vi "newposition.vi"(0 "x_modify":dbl, 4 "cur_y":dbl, 5 "r":dbl, 6 "cur_x":dbl, 7 "y_modify":dbl, 8 "dt":dbl=0.02, 9 "V_right":dbl, 10 "V_left":dbl, 11 "cur_angle":dbl) -> (1 "new_y":dbl, 2 "new_x":dbl, 3 "new_angle":dbl)   [LabVIEW 2015]
uses:
  Documents/LabVIEW Data/MathScriptVIs/MCStatic_35241984432_abfa35976836e38269e549687f4c5e7d.vi
  <instcachedir>/0/MCStatic_35241984432_abfa35976836e38269e549687f4c5e7d_C7C269247EEA4349BB5C711C73CDF5A1.lvgen/MCStatic_35241984432_abfa35976836e38269e549687f4c5e7d_C7C269247EEA4349BB5C711C73CDF5A1_000.vi
  <vilib>/imath/engines/lvmath2/RunTimeEngine/NodeEndStatement/NIMS_NodeEndStatement_Output.vi
  <instcachedir>/0/NIMS_NodeEndStatement_Output_53EC0D466D134D7ABD903AC30B43404B.lvgen/NIMS_NodeEndStatement_Output_53EC0D466D134D7ABD903AC30B43404B_001.vi
  <vilib>/imath/engines/lvmath2/RunTimeEngine/ErrorHandling/NIMS_Finalize Error.vi
  Documents/LabVIEW Data/Coordinates.m
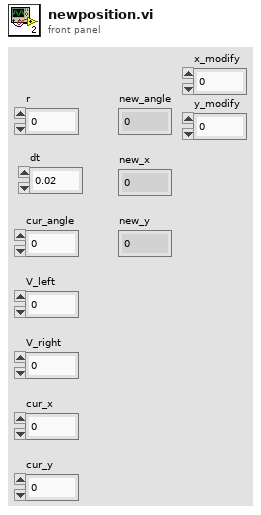
[diagram p1: front panel]
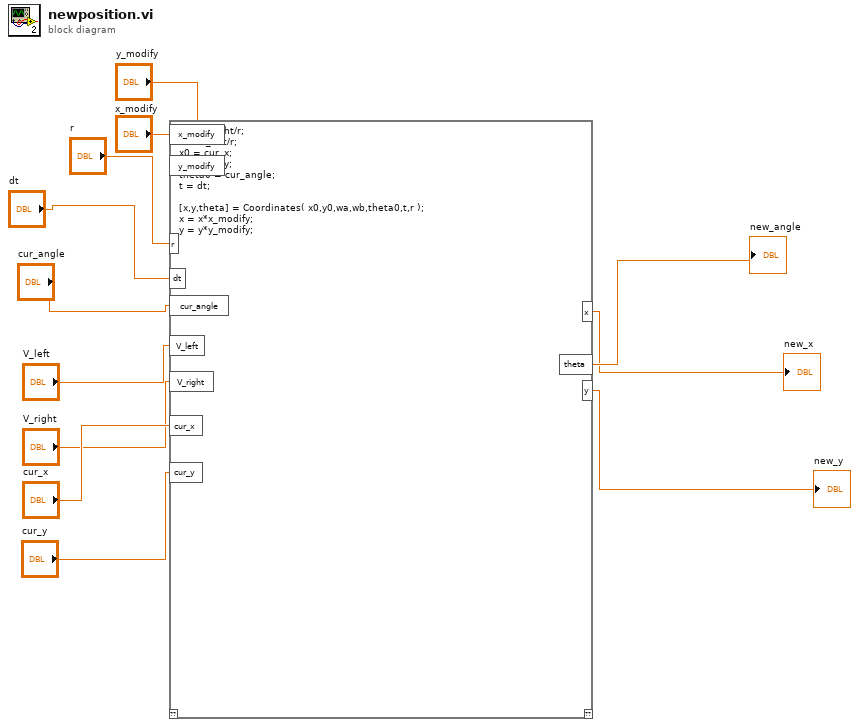
[diagram p0: block diagram]
diagram:
  n1 = mathscript code="wa=V_right/r;\nwb=V_left/r;\nx0 = cur_x;\ny0 = cur_y;\ntheta0 = cur_angle;\nt = dt;\n\n[x,y,theta] = Coordinates( x0,y0,wa,wb,theta0,t,r );\nx = x*x_modify;\ny = y*y_modify;"("dt"="dt", "cur_angle"="cur_angle", "V_left"="V_left", "V_right"="V_right", "cur_x"="cur_x", "cur_y"="cur_y", "r"="r", "x_modify"="x_modify", "y_modify"="y_modify") -> ("x"=→"new_x":dbl, "theta"=→"new_angle":dbl, "y"=→"new_y":dbl)  [unwired: 1 in, 1 out]
